vi "Get Available Pixel Formats.vi"(8 "error in (no error)":errorcluster, 11 "Camera in":refnum<class "Camera.lvclass">) -> (0 "error out":errorcluster, 2 "Pixel Formats":string[](array[string]), 3 "Camera":refnum<class "Camera.lvclass">)   [LabVIEW 2020, in "Camera.lvclass"]
uses:
  Camera.lvclass
  Camera.lvclass/Camera.ctl
  bin/gindustrialcam_32-1.dll
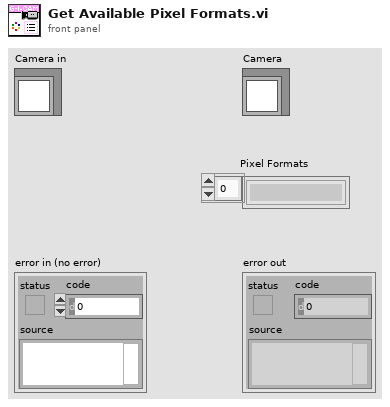
[diagram p1: front panel]
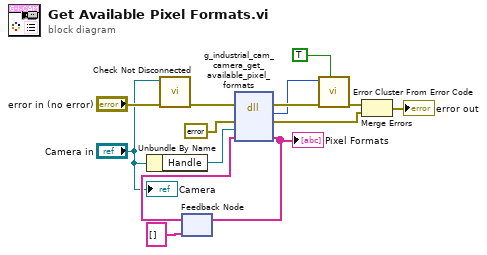
[diagram p0: block diagram]
diagram:
  n1 = Unbundle By Name("Camera in") -> ("Handle"=w3:refnum<data-value>)
  n2 = call "Check Not Disconnected.vi"("error in (no error)"="error in (no error)", "Camera in"="Camera in") -> ("error out"=w2:errorcluster)  [unwired: 9 in]
  n3 = feedback #1(string[] []) -> (w5:string[])
  n4 = dll-call lib="C:/serenial/lib/g-industrial-camera/LabVIEW/g_industrial_cam/bin/gindustrialcam_*-1.*" fn="g_industrial_cam_camera_get_available_pixel_formats"(error in=w2, "err"=errorcluster {"status"=FALSE, "code"=0, "source"=""} ("error constant"), "edvr"=w3, "formats"=w5) -> (error out=w12:errorcluster, "Mg_Error"=w11:i32, "err"=w9:errorcluster, "formats"=w4:string[])  [unwired: 3 in, 1 out]
  "Pixel Formats" <- w4
  n5 = feedback-in #1(w4) -> ()
  n6 = call <vilib>:"Error Cluster From Error Code.vi"("show call chain? (False)"=TRUE, "error in (no error)"=w12, "error code (0)"=w11) -> ("error out"=w10:errorcluster)  [unwired: 6 in]
  n7 = Merge Errors(w10, w9) -> (→"error out":errorcluster)
  "Camera" <- "Camera in"
